vi "CRYGet Step Name Dialog.vi"(10 "Step Name":string caption="µÑ\\¸tÇ„¹DÇ …Ç%¸XÕíÂÜÂ$Æ.") -> (2 "Step Name Out":string, 3 "Return Flag":bool)   [LabVIEW 2013]
panel:
  in  "Cancel":bool
  in  "OK":bool
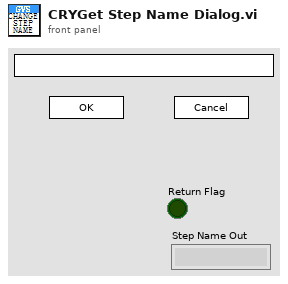
[diagram p1: front panel]
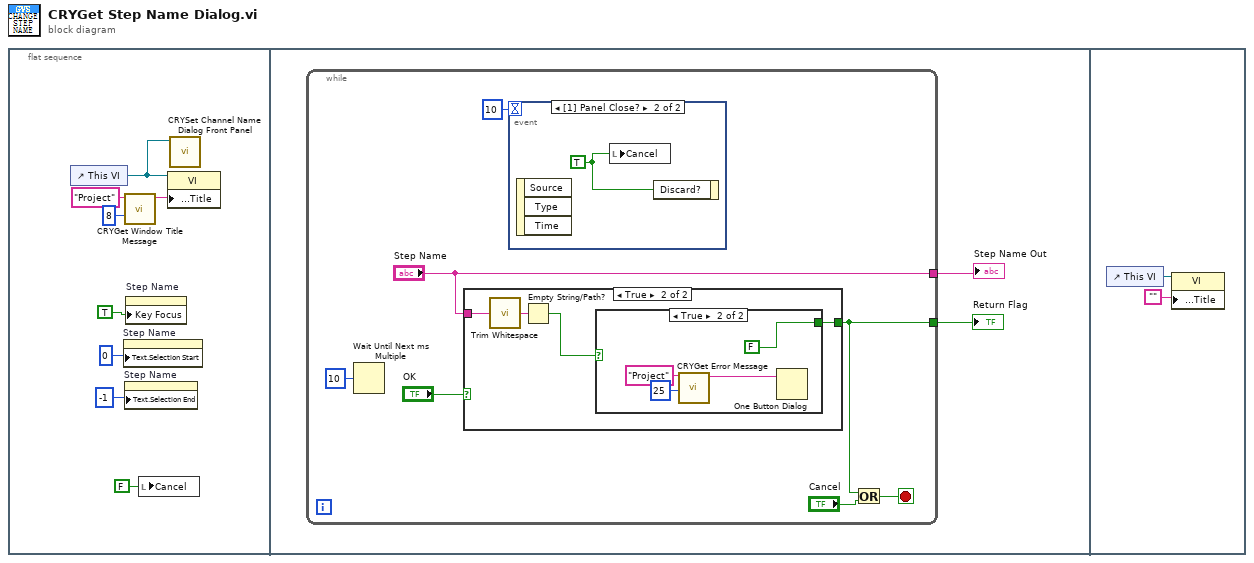
[diagram p0: block diagram]
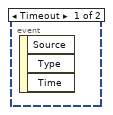
[diagram p2: hidden frame]
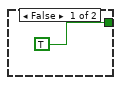
[diagram p4: hidden frame]
diagram:
  n1 = flat-sequence {
    frame #0 {
      n2 = control-ref of="This VI"() -> (w5:refnum<vi>)
      n3 = property on="Step Name" class="Str"("Text.Selection Start"=u32 0 ("Text.Selection:Start")) -> ()  [unwired: 2 in, 2 out]
      n4 = call "CRYGet Window Title Message.vi"("No"=8 ("Error No"), "Kind"="Project") -> ("Multibyte String"=w1:string)  [unwired: 4 in, 5 out]
      n5 = property on="Step Name" class="Str"("Text.Selection End"=-1 ("Text.Selection:End")) -> ()  [unwired: 2 in, 2 out]
      n6 = property on="Step Name" class="Str"("Key Focus"=TRUE) -> ()  [unwired: 2 in, 2 out]
      n7 = local write "Cancel"(FALSE ("Cancel")) -> ()
      n8 = property class="VI"(reference=w5, "Front Panel.Title"=w1) -> ()  [unwired: 1 in, 2 out]
      n9 = call "CRYSet Channel Name Dialog Front Panel.vi"("Vi Ref"=w5) -> ()  [unwired: 11 in]
    }
    frame #1 {
      n10 = while {
        tunnel: ["Step Name"] -> w10
        tunnel: [w12] -> w9
        stop <- w17 stop-if-true
        n11 = Wait Until Next ms Multiple(millisecond multiple=u32 10) -> ()  [unwired: 1 out]
        n12 = case shown="True" "OK" {
          selector: "OK" -> [w19 _]
          tunnel: [w19 w21] -> w12
          tunnel: "Step Name" -> [_ w23]
          frame False {
          }
          frame True {
            n13 = call <vilib>:"Trim Whitespace.vi"("string"=w23) -> ("trimmed string"=w20:string)  [unwired: 1 in]
            n14 = Empty String/Path?(string/path=w20) -> (empty?=w22:bool)
            n15 = case shown="True" w22 {
              tunnel: [TRUE ("empty?") FALSE ("empty?")] -> w21
              frame False {
              }
              frame True {
                n16 = call "CRYGet Error Message.vi"("Error No"=25 ("No"), "Kind"="Project") -> ("Message"=w25:string)  [unwired: 4 in, 5 out]
                n17 = One Button Dialog(message=w25) -> ()  [unwired: 2 out]
              }
            }
          }
        }
        n18 = event shown="[1] Panel Close?" {
          selector: _ -> [_ _]
          dyn-events: _ -> [_ _]
          timeout: 10 -> [_ _]
          event Timeout {
            n19 = event-data() -> ()  [unwired: 1 in, 3 out]
          }
          event Panel Close? {
            w18 = TRUE ("OK")
            n20 = event-data() -> ()  [unwired: 1 in, 3 out]
            n21 = local write "Cancel"(w18) -> ()
            n22 = event-data("Discard?"=w18) -> ()  [unwired: 1 in, 1 out]
          }
        }
        n23 = Or(x=w12, y="Cancel") -> (x .or. y?=w17:bool)
      }
      "Return Flag" <- w9
      "Step Name Out" <- w10
    }
    frame #2 {
      n24 = control-ref of="This VI"() -> (w30:refnum<vi>)
      n25 = property class="VI"(reference=w30, "Front Panel.Title"="") -> ()  [unwired: 1 in, 2 out]
    }
  }
